vi "Write Destination path.vi"(10 "Destination path":path, 11 "ProjectItem in":refnum<class "ProjectItem.lvclass">) -> (3 "ProjectItem out":refnum<class "ProjectItem.lvclass">)   [LabVIEW 2019, in "SolutionBuilder.lvlib" / "ProjectItem.lvclass"]
uses:
  ProjectItem.lvclass
  ProjectItem.lvclass/ProjectItem.ctl
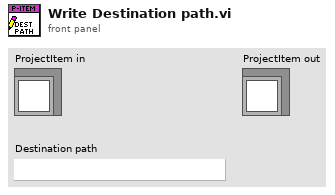
[diagram p1: front panel]
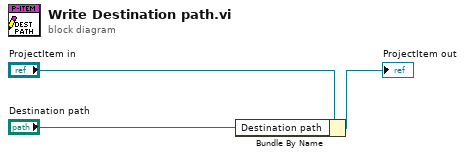
[diagram p0: block diagram]
diagram:
  n1 = Bundle By Name(cluster="ProjectItem in", "Destination path"="Destination path") -> (→"ProjectItem out":refnum<class "ProjectItem.lvclass">)
